vi "ProbePlanParams.vi"() -> ()   [LabVIEW 2018]
doc: "Global variable with information about the layout of the DUT."
panel:
  out "ProbePlan Parameters IN":T1 {"ProbePlan array"."ProbePoints"."Y" format="%_2g"; "ProbePlan array"."ProbePoints"."X" format="%_2g"; "Relative strip angles" format="%.6f"; "Radius" format="%.2f"; "Fiducail separation" format="%.2f"; "Strip pitch" format="%.2f"; "Yoffset" format="%.2f"; "Device Orientation" format="%.6f"; "l_outer" format="%.6f"; "l_inner" format="%.6f"; "Outer pads offset" format="%.6f"; "Inner pads offset" format="%.6f"}
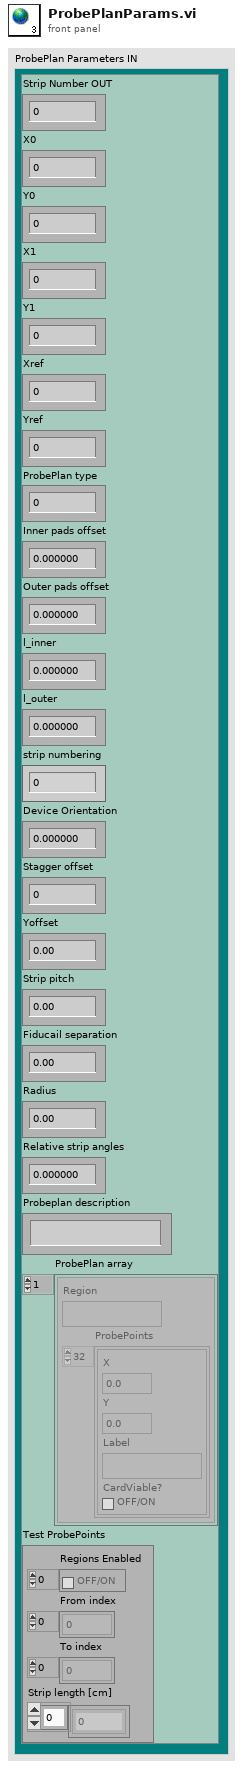
[diagram p1: front panel]
types:
  T1 = cluster{"Strip Number OUT":i32, "X0":i32, "Y0":i32, "X1":i32, "Y1":i32, "Xref":dbl, "Yref":dbl, "ProbePlan type":u32, "Inner pads offset":ext, "Outer pads offset":ext, "l_inner":ext, "l_outer":ext, "strip numbering":u16, "Device Orientation":ext, "Stagger offset":i32, "Yoffset":dbl, "Strip pitch":dbl, "Fiducail separation":dbl, "Radius":ext, "Relative strip angles":dbl, "Probeplan description":string, "ProbePlan array":cluster{"Region":string, "ProbePoints":cluster{"X":dbl, "Y":dbl, "Label":string, "CardViable?":bool}[]}[], "Test ProbePoints":cluster{"Regions Enabled":bool[], "From index":u32[], "To index":u32[], "Strip length [cm]":dbl[]}}
diagram:
